vi "Pre Launch Init.vi"(11 "Child_1 in":refnum<class "Child_2_Class.lvclass">=refnum) -> (0 "error out":errorcluster, 3 "Child_1 out":refnum<class "Child_2_Class.lvclass">)   [LabVIEW 2023, in "Actor_Child_2.lvlib" / "Child_2_Class.lvclass"]
doc: "(<B>Filename</B>: Actor Framework.lvlib:Actor.lvclass:Pre Launch Init.vi)\n\nDefines behavior that occurs after the Launch Nested Actor method is invoked but before the actor's Actor Core method begins running.\n\nBy default, this method does nothing. A descendant class may override it to define behavior."
uses:
  Child_2_Class.lvclass
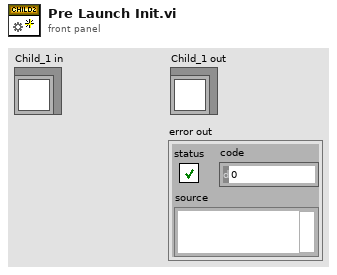
[diagram p1: front panel]
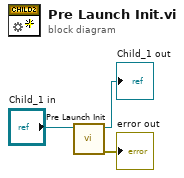
[diagram p0: block diagram]
diagram:
  n1 = call-parent "Pre Launch Init.vi"("Actor in"="Child_1 in") -> ("error out"=→"error out":errorcluster, "Actor out"=→"Child_1 out":refnum<class "Child_2_Class.lvclass">)  [unwired: 9 in]
